vi "FringeTrackerGUI.vi"() -> ()   [LabVIEW 2009, in "FringeTracker.lvlib"]
uses:
  FringeTracker.lvlib
  Controls/FringeTrackerInfo.ctl
  Nicmos/Controls/NICMOS.READOUT.ctl
  Controls/FringeTrackerState.ctl
  Controls/FringeTrackerData.ctl
panel:
  out "State":T1
  in  "Frame per fringe":dbl=5.0
  in  "Autcollimation":bool
  in  "Wavelength":dbl[unit]=1.3e-06
  in  "Readout":T2={"Readout"=512, "Deglitch"=30, "Framerate"=2000.0, "Bank"=2}
  out "FringeTrackerInfo":T3={"Readout"={"Readout"=100, "Deglitch"=10, "Framerate"=200.0, "Bank"=2}, "OPD stroke"=0.0, "OPD per pixel"=0.0}
  in  "IDLE Button":bool
  in  "SCAN Button":bool
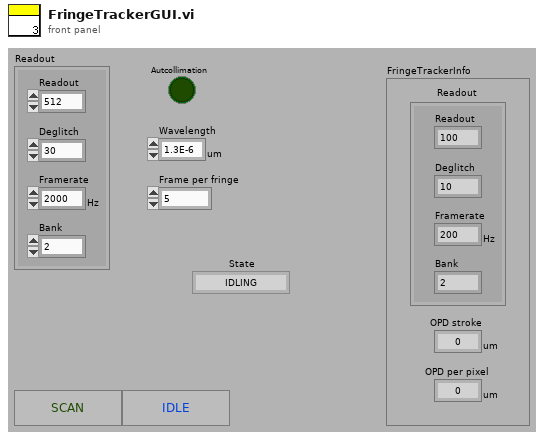
[diagram p1: front panel]
types:
  T1 = typedef "FringeTrackerState.ctl" = enum16{"IDLING", "CONFIGURING", "SCANNING", "SEARCHING", "TRACKING", "STOPPING"}
  T2 = typedef "NICMOS.READOUT.ctl" = cluster{"Readout":i32, "Deglitch":i32, "Framerate":dbl[unit], "Bank":i32}
  T3 = typedef "FringeTrackerInfo.ctl" = cluster{"Readout":T2, "OPD stroke":dbl[unit], "OPD per pixel":dbl[unit]}
  T4 = typedef "FringeTrackerData.ctl" = cluster{"Readout":T2, "Wavelength":dbl[unit], "Frame per fringe":dbl, "Autcollimation":bool, "OPD stroke":dbl[unit], "OPD per pixel":dbl[unit], "Offset":dbl[unit]}
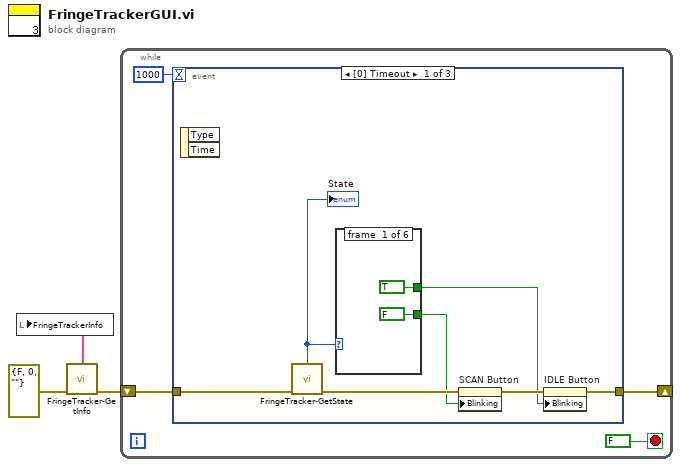
[diagram p0: block diagram]
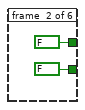
[diagram p2: hidden frame]
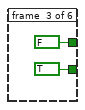
[diagram p3: hidden frame]
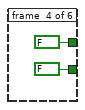
[diagram p4: hidden frame]
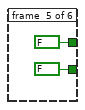
[diagram p5: hidden frame]
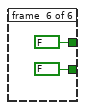
[diagram p6: hidden frame]
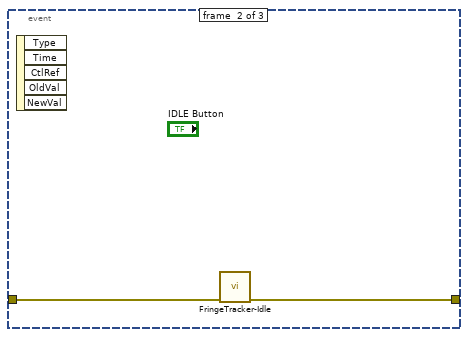
[diagram p7: hidden frame]
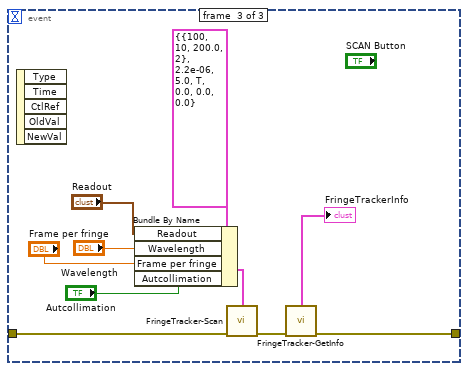
[diagram p8: hidden frame]
diagram:
  n1 = call "FringeTracker-GetInfo.vi"("error in (no error)"=errorcluster {"status"=FALSE, "code"=0, "source"=""} ("error out")) -> ("FringeTrackerInfo"=w1:T3, "error out"=w2:errorcluster)  [unwired: 7 in]
  n2 = local write "FringeTrackerInfo"(w1) -> ()
  n3 = while {
    shift-right: [w6] -> _
    shift-left: w2 -> [w7]
    stop <- FALSE stop-if-true
    n4 = event shown="[0] Timeout" {
      selector: _ -> [_ _ _]
      dyn-events: _ -> [_ _ _]
      timeout: 1000 -> [_ _ _]
      tunnel: w7 -> [w8 w28 w38]
      tunnel: [w11 w27 w30] -> w6
      event #0 {
        n5 = event-data() -> ()  [unwired: 1 in, 2 out]
        n6 = call "FringeTracker-GetState.vi"("error in (no error)"=w8) -> ("State"=w14:T1, "error out"=w12:errorcluster)  [unwired: 7 in]
        "State" <- w14
        n7 = case shown="\"IDLING\", Default" w14 {
          tunnel: [TRUE FALSE FALSE FALSE FALSE FALSE] -> w10
          tunnel: [FALSE FALSE TRUE FALSE FALSE FALSE] -> w9
          frame #0 {
          }
          frame #1 {
          }
          frame #2 {
          }
          frame #3 {
          }
          frame #4 {
          }
          frame #5 {
          }
        }
        n8 = property on="SCAN Button" class="Bool"(error in=w12, "Blinking"=w9) -> (error out=w13:errorcluster)  [unwired: 1 in, 1 out]
        n9 = property on="IDLE Button" class="Bool"(error in=w13, "Blinking"=w10) -> (error out=w11:errorcluster)  [unwired: 1 in, 1 out]
      }
      event #1 {
        n10 = event-data() -> ()  [unwired: 1 in, 5 out]
        n11 = call "FringeTracker-Idle.vi"("error in (no error)"=w28) -> ("error out"=w27:errorcluster)  [unwired: 10 in]
      }
      event #2 {
        n12 = event-data() -> ()  [unwired: 1 in, 5 out]
        n13 = Bundle By Name(cluster=T4 {"Readout"={"Readout"=100, "Deglitch"=10, "Framerate"=200.0, "Bank"=2}, "Wavelength"=2.2e-06, "Frame per fringe"=5.0, "Autcollimation"=TRUE, "OPD stroke"=0.0, "OPD per pixel"=0.0, "Offset"=0.0} ("FringeTrackerData"), "Readout"="Readout", "Wavelength"="Wavelength", "Frame per fringe"="Frame per fringe", "Autcollimation"="Autcollimation") -> (w36:T4)
        n14 = call "FringeTracker-Scan.vi"("FringeTrackerData"=w36, "error in (no error)"=w38) -> ("error out"=w31:errorcluster)  [unwired: 7 in]
        n15 = call "FringeTracker-GetInfo.vi"("error in (no error)"=w31) -> ("FringeTrackerInfo"=→"FringeTrackerInfo":T3, "error out"=w30:errorcluster)  [unwired: 7 in]
      }
    }
  }
